vi "Surface Page.vi"() -> ()   [LabVIEW 2020, in "3D Surface.lvclass"]
uses:
  <vilib>/Math Plots/3D Math Plots/3D Surface/3D Surface/3D Surface.lvclass
  <vilib>/Math Plots/3D Math Plots/3D Surface/3D Surface/Typedef/3D Surface Property Array.ctl
  <vilib>/Math Plots/3D Math Plots/3D Surface/3D Surface/Typedef/3D Surface Property.ctl
  <vilib>/Math Plots/3D Math Plots/3D Plot/3D Plot/Typedef/Color Ramp Cluster.ctl
  <vilib>/Math Plots/3D Math Plots/3D Plot/3D Plot/Typedef/Line Type.ctl
  <vilib>/Math Plots/3D Math Plots/3D Plot/3D Plot/Typedef/Dialog State.ctl
  <vilib>/Math Plots/3D Math Plots/3D Plot/3D Plot/Typedef/Temp Scene State.ctl
  <vilib>/Math Plots/3D Math Plots/3D Plot/3D Plot/Typedef/Temp Scene Property Action.ctl
  <vilib>/Math Plots/3D Math Plots/3D Plot/3D Plot/3D Plot.lvclass
panel:
  in  "Draw Normal":bool caption="Draw surface"
  in  "Draw Mesh":bool caption="Draw surface"
  in  "Color Mode":u16(ring) caption="Color mode" items=["Flat Shading", "Interpolated Shading"]
  in  "Antialiasing":bool
  in  "Line Color":u32(colorbox) caption="Line color"
  in  "Line Width":sgl=0.001 caption="Line width" min=0.001 step=1
  in  "Line Style":u16(ring) caption="Line style"
  in  "Draw Surface":bool caption="Draw surface"
  out "Surface Property Out":T1
  in  "Surface Property In":T1
  out "Color Ramp":dbl[][](graph)
  in  "Color Map Style":u16(ring) caption="Color map style" items=["None ", "Shaded", "Color spectrum", "Grey scale", "Custom"]
  in  "YZ Plane Projection":bool caption="YZ plane projection"
  in  "XZ Plane Projection":bool caption="XZ plane projection"
  in  "XY Plane Projection":bool caption="XY plane projection"
  in  "Coordinate System":u16(ring) caption="Coordinate system" items=["Cartesian", "Cylindrical", "Spherical"]
  in  "Plot Opacity":sgl(slide) caption="Plot opacity(%)" min=0 max=100 scale=0.0..100.0
  in  "Plot List":i32(listbox)
  in  "Ramp Edit":bool caption="Ramp edit"
  in  "Move Down":bool
  in  "Move Up":bool
  in  "Delete":bool
  in  "New":bool
  in  "Event Registration":refnum<event-registration>
  # "Surface"
  # "General"
  # "Projection"
  # "Color Ramp"
  # "Surface"
  # "Mesh"
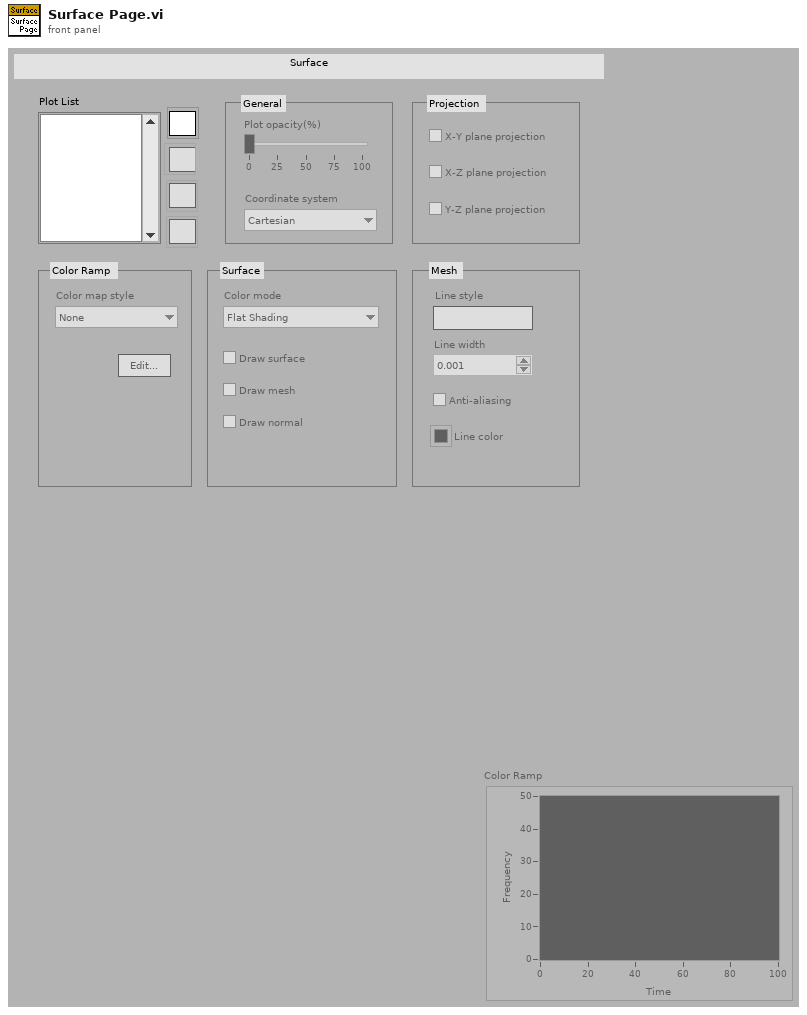
[diagram p1: front panel]
types:
  T1 = typedef "3D Surface.lvclass/3D Surface Property Array.ctl" = T2[]
  T2 = typedef "3D Surface.lvclass/3D Surface Property.ctl" = cluster{"General Property":cluster{"Plot Name":string, "Coordinate System":enum16{"Cartesian", "Cylindrical", "Spherical"}, "Opacity":sgl}, "Projection Property":cluster{"Draw XY":bool, "Draw YZ":bool, "Draw XZ":bool}, "Plot Property":cluster{"Draw Surface":bool, "Draw Mesh":bool, "Draw Normal":bool, "Color Ramp Cluster":T3, "Line Style":T4, "Line Width":sgl, "Line Color":u32, "Antialiasing":bool}, "Surface Property":cluster{"Color Mode":enum16{"Flat Shading", "Interpolated Shading"}}}
  T3 = typedef "3D Plot.lvclass/Color Ramp Cluster.ctl" = cluster{"Color Ramp Style":enum16{"None", "Shaded", "Color spectrum", "Grey scale", "Custom"}, "Color Ramp Array":u32[], "Color Ramp Index":i32[], "Interpolate?":bool, "Logarithm?":bool}
  T4 = typedef "3D Plot.lvclass/Line Type.ctl" = enum16{"None", "Solid", "Dash", "Dot", "Dash Dot"}
  T5 = typedef "3D Plot.lvclass/Dialog State.ctl" = enum16{"Initialize", "Read Porperty", "Write Property", "Idle", "Exit"}
  T6 = typedef "3D Plot.lvclass/Temp Scene State.ctl" = enum16{"Create", "Update Scene", "Get Plot Representation", "Destory"}
  T7 = typedef "3D Plot.lvclass/Temp Scene Property Action.ctl" = enum16{"Graph Property", "Light Property", "Axis Property", "Value Pair Property", "Format Property", "Cursor Property", "Plot Specific Property"}
  T8 = typedef "3D Plot.lvclass/Multiplot Representation.ctl" = cluster{"Plot Represention Array":T9[], "Max Range":T10}
  T9 = typedef "3D Plot.lvclass/Plot Representation.ctl" = cluster{"Plot ID":i32, "Plot Range":T10, "Mesh Data":T11, "Dimension":cluster{"X Dimension":i32, "Y Dimension":i32}, "Ramp Range":T10}
  T10 = typedef "3D Plot.lvclass/Range Clusters.ctl" = cluster{"X Range":cluster{"Max X":sgl, "Min X":sgl}, "Y Range":cluster{"Max Y":sgl, "Min Y":sgl}, "Z Range":cluster{"Max Z":sgl, "Min Z":sgl}}
  T11 = typedef "3D Plot.lvclass/Mesh Data.ctl" = cluster{"Index Array":u32[], "Vertex Array":cluster{"X":sgl, "Y":sgl, "Z":sgl}[], "Normal Array":cluster{"X":sgl, "Y":sgl, "Z":sgl}[], "Color Index Array":i32[]}
  T12 = enum16{"None", "Shaded", "Color spectrum", "Grey scale", "Custom"}
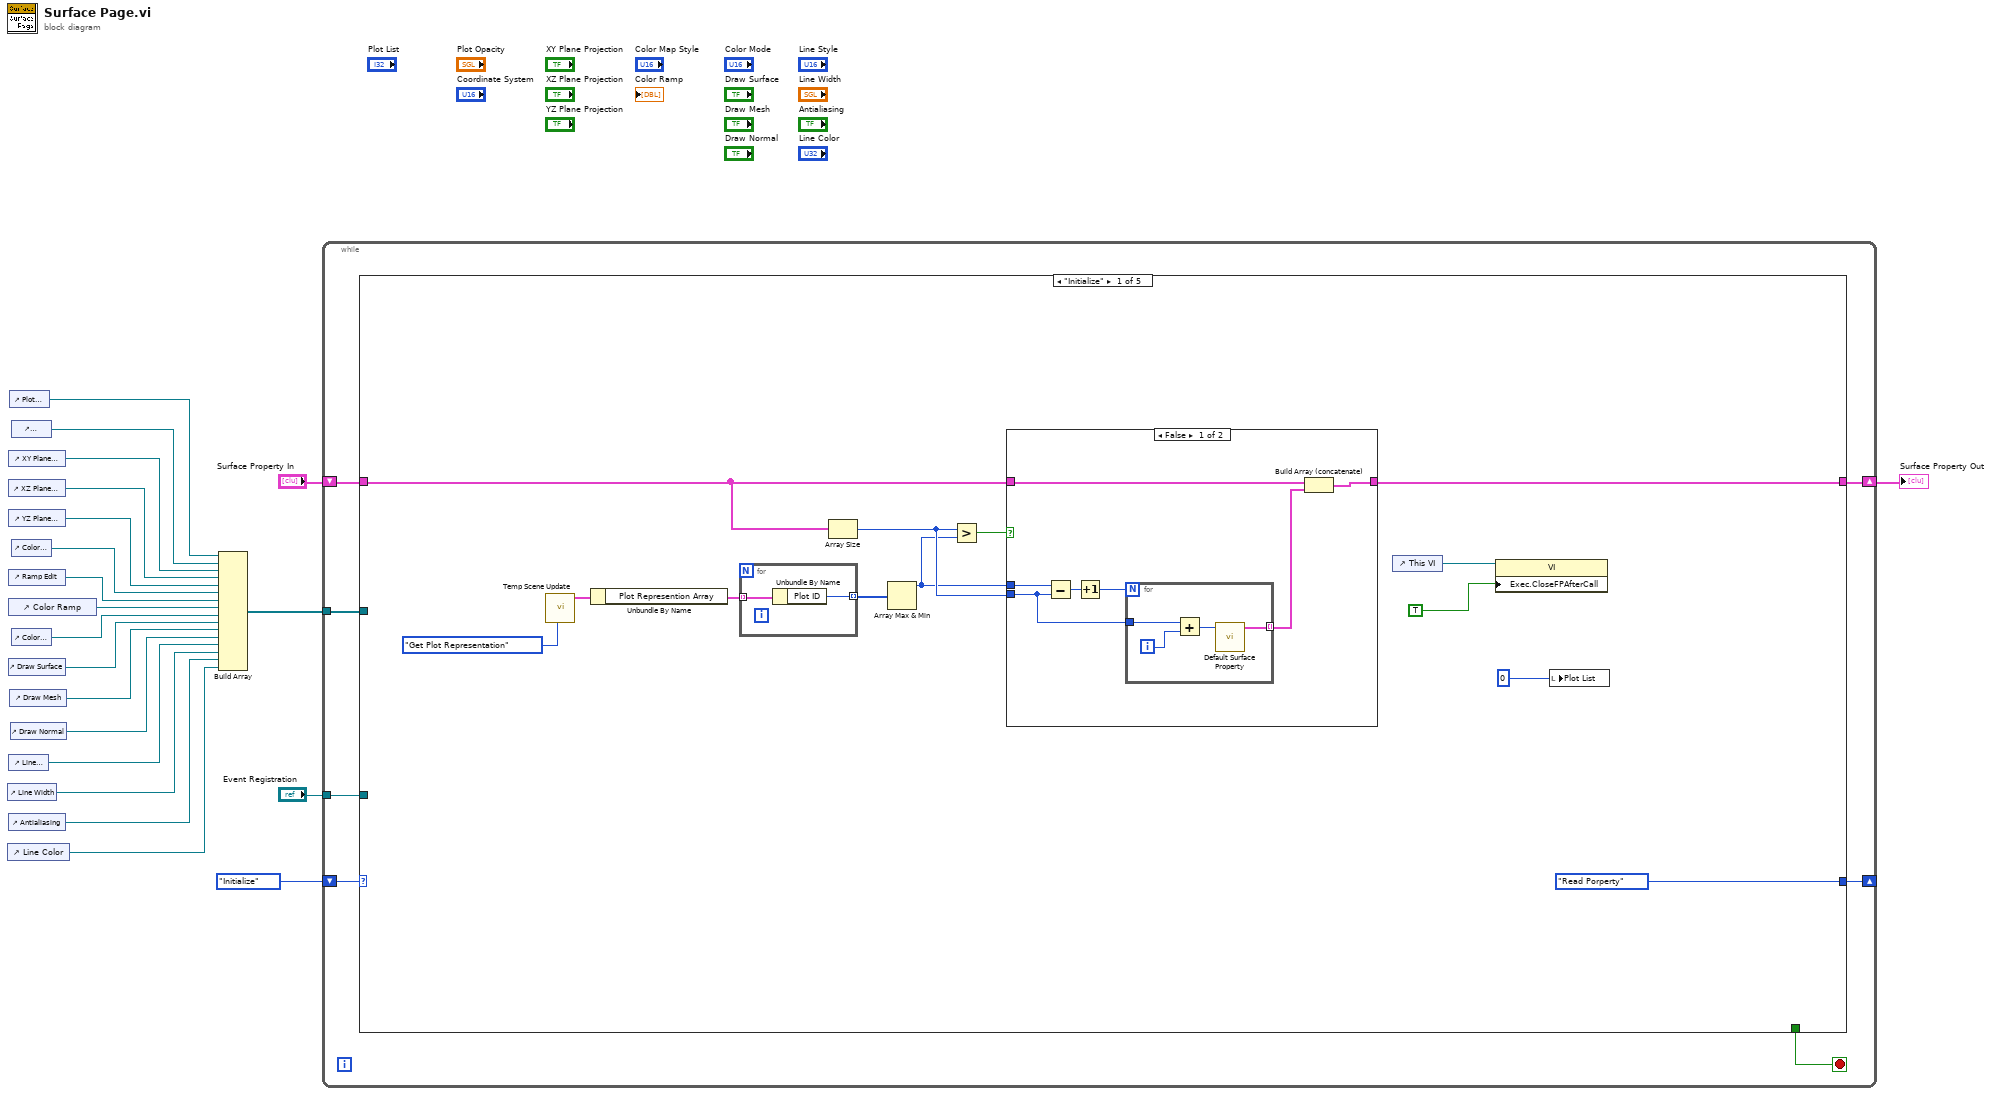
[diagram p0: block diagram]
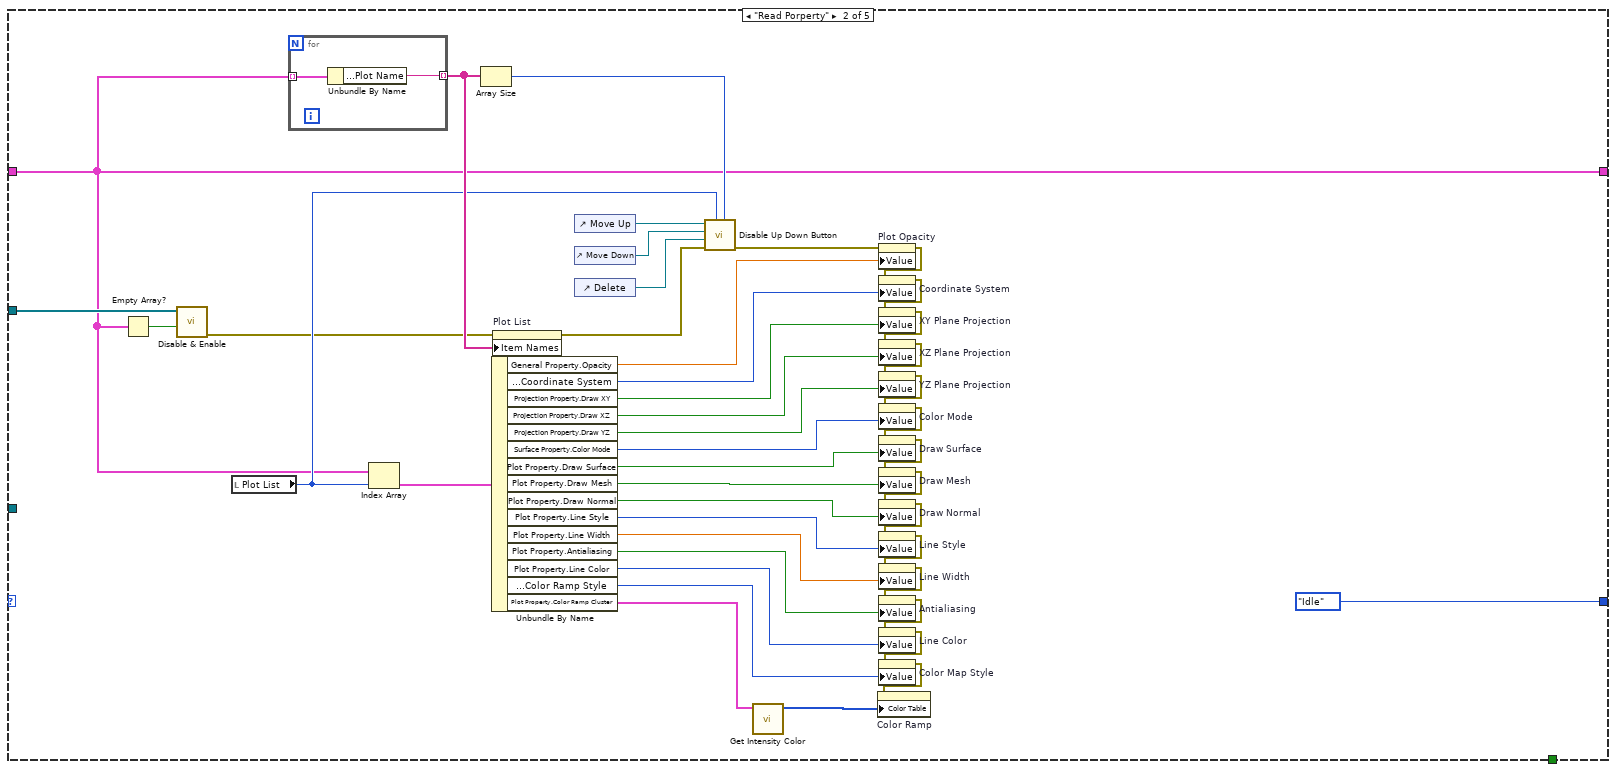
[diagram p3: hidden frame]
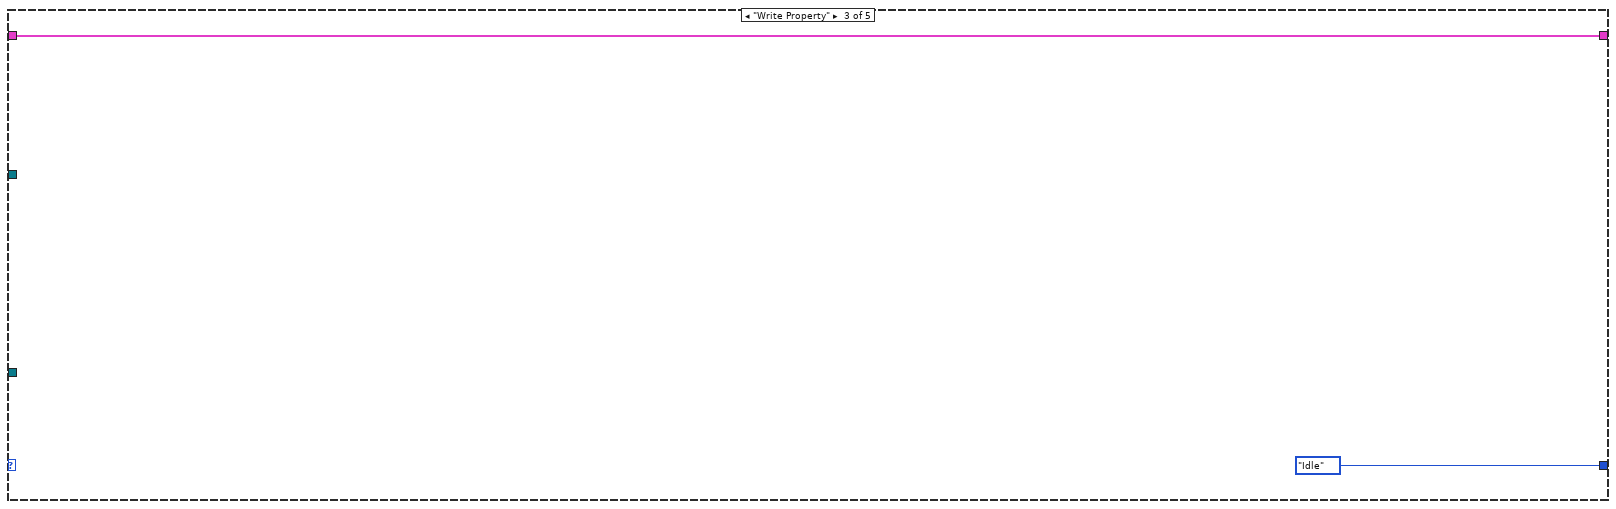
[diagram p4: hidden frame]
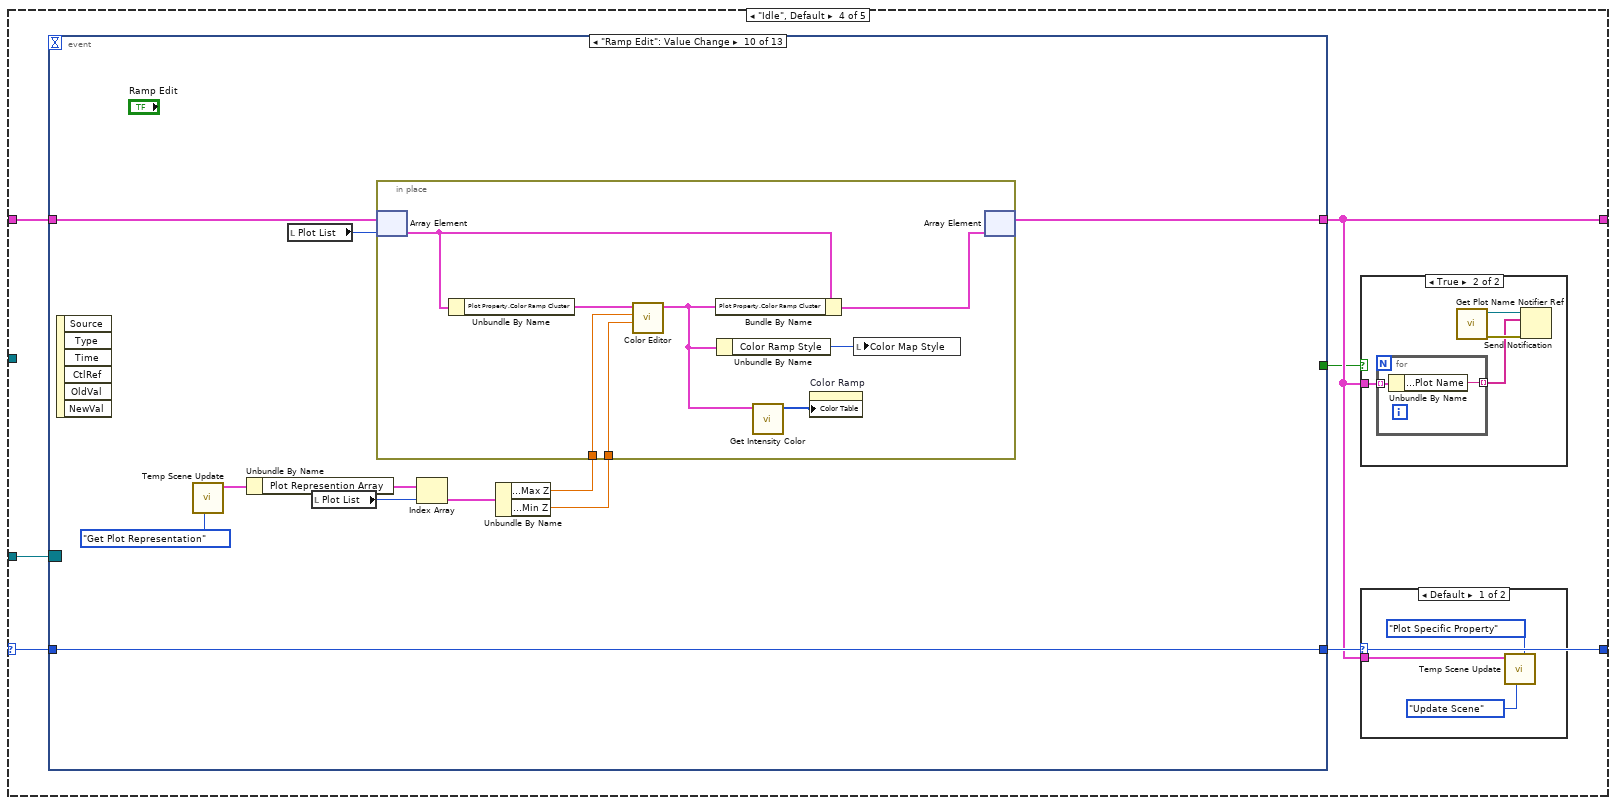
[diagram p5: hidden frame]
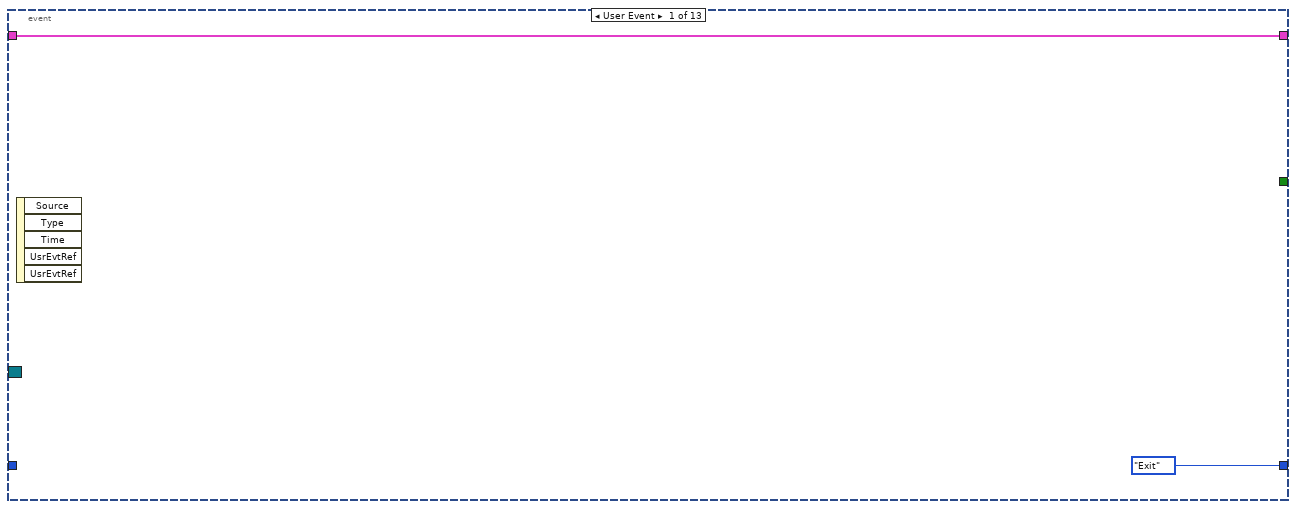
[diagram p8: hidden frame]
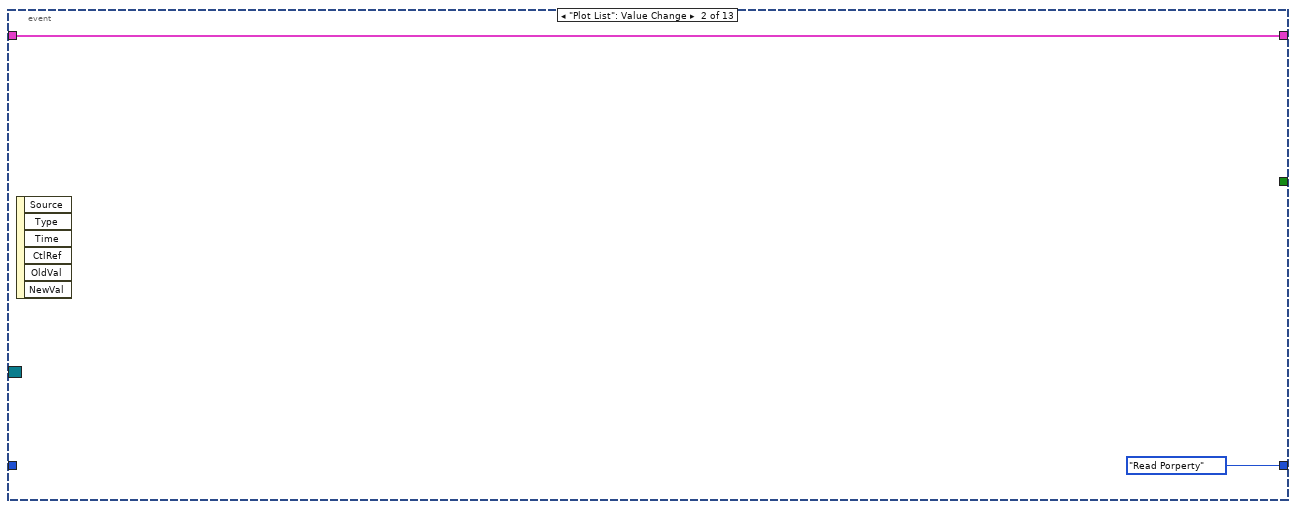
[diagram p9: hidden frame]
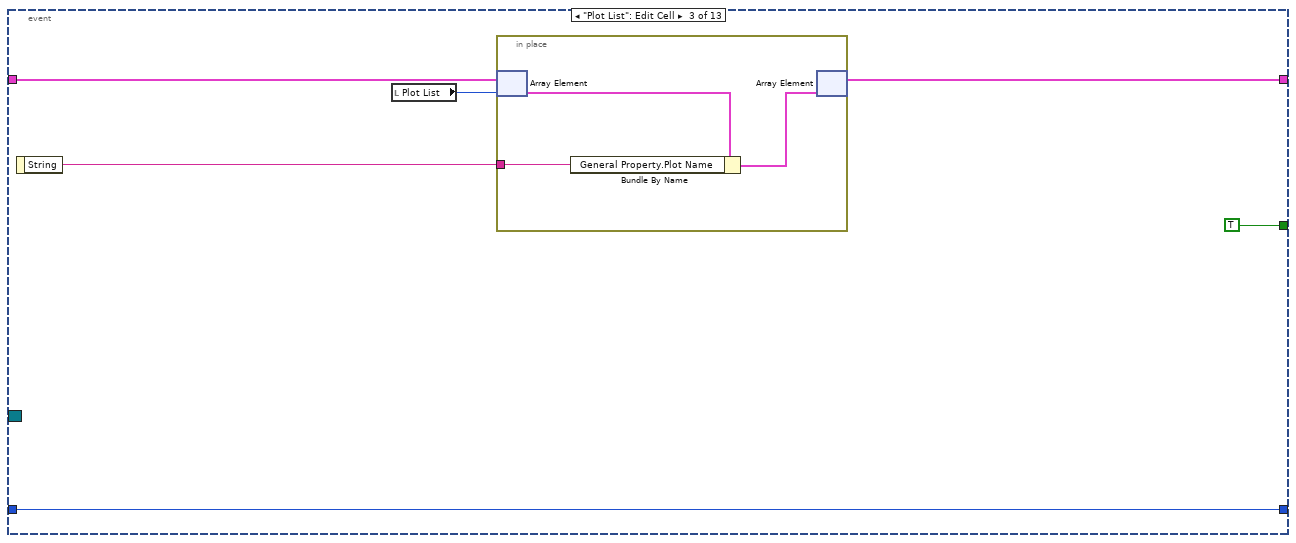
[diagram p10: hidden frame]
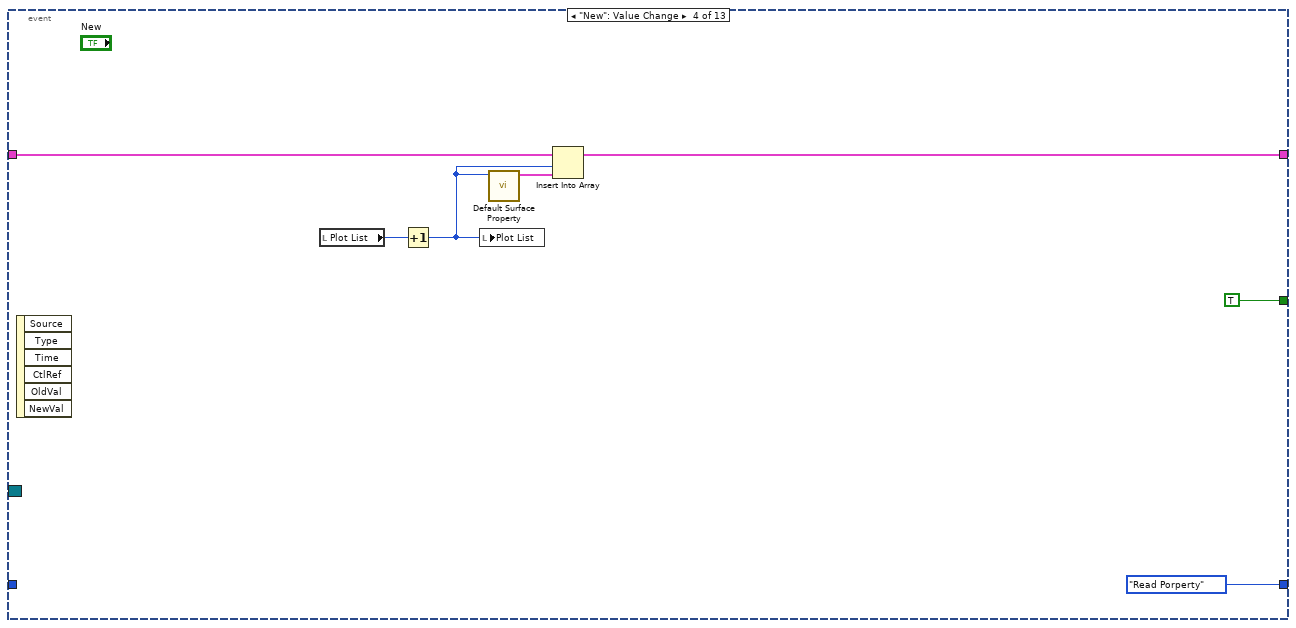
[diagram p11: hidden frame]
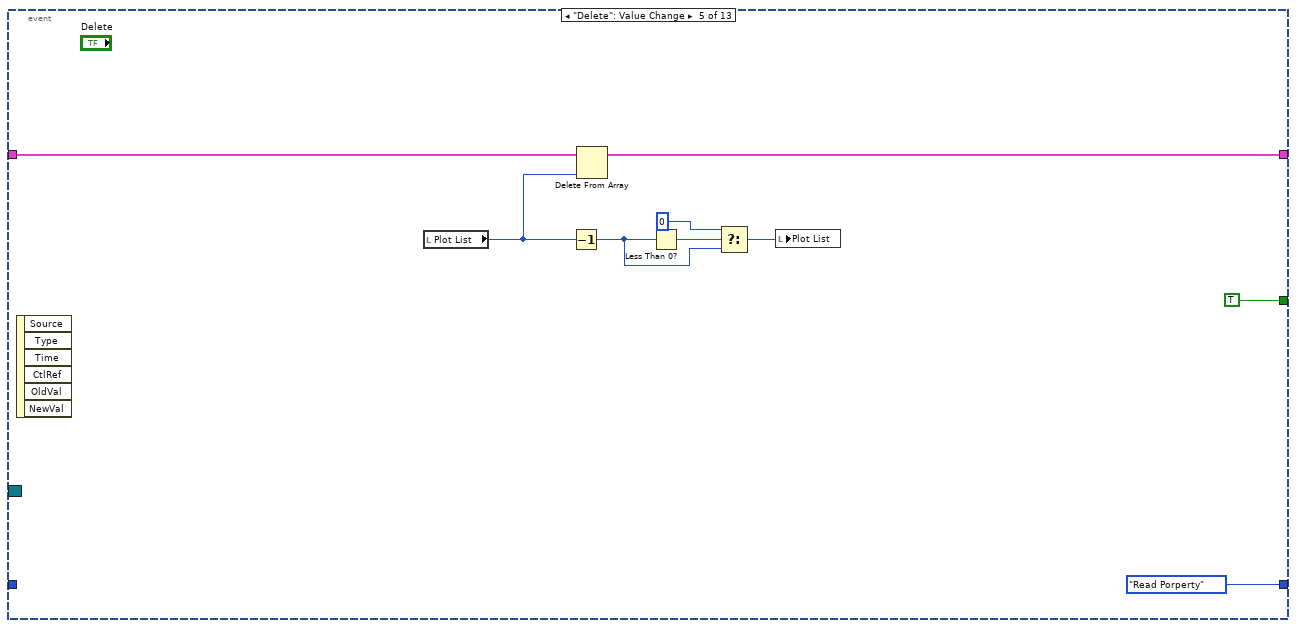
[diagram p12: hidden frame]
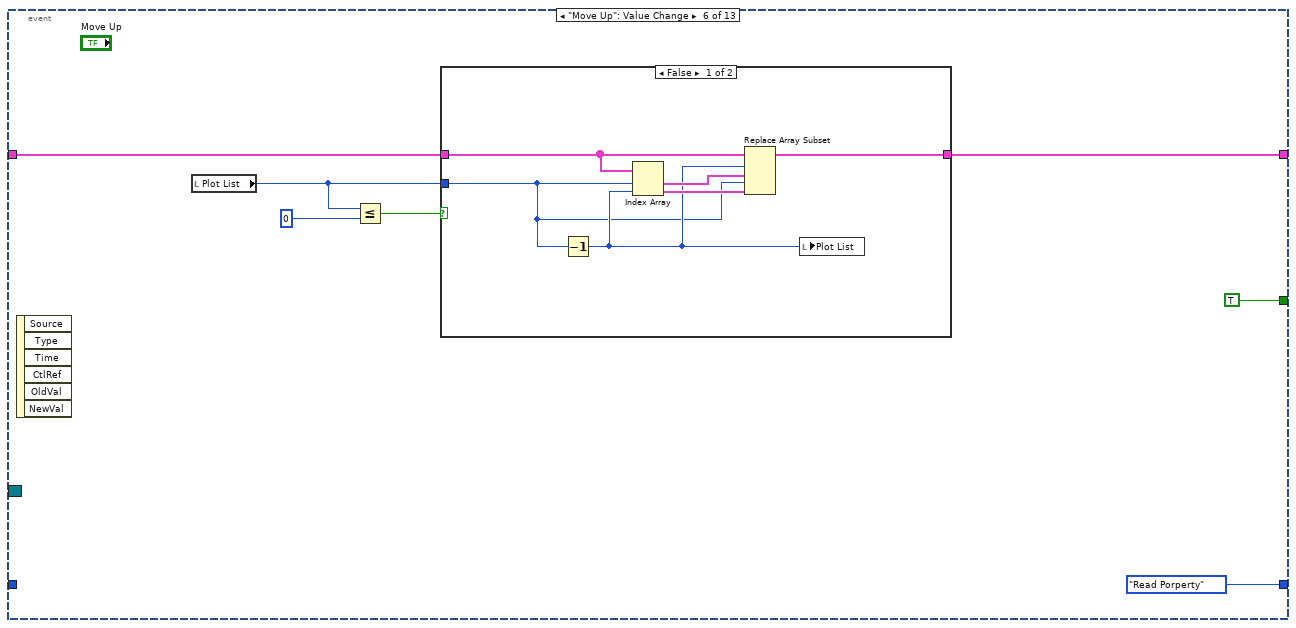
[diagram p13: hidden frame]
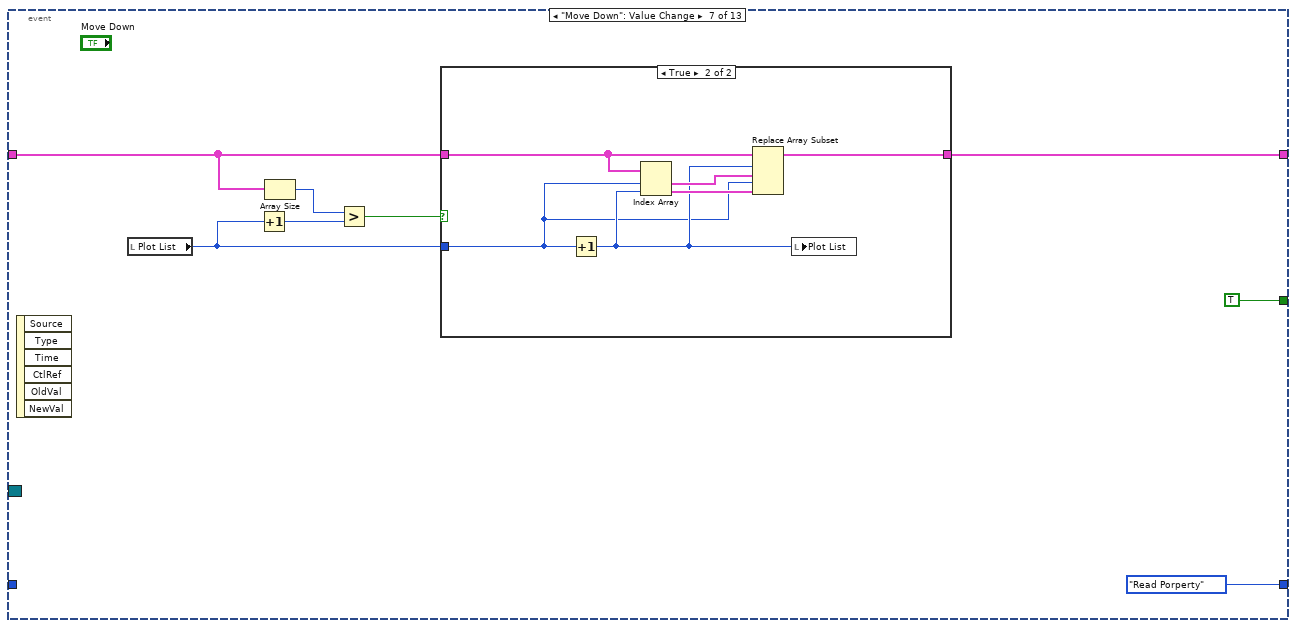
[diagram p15: hidden frame]
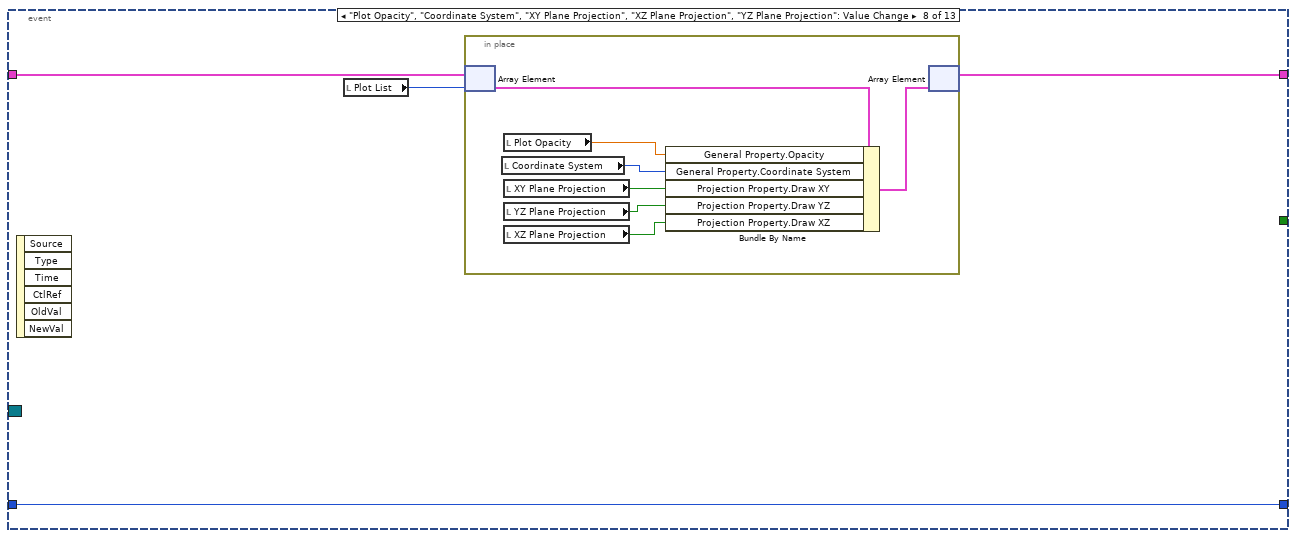
[diagram p17: hidden frame]
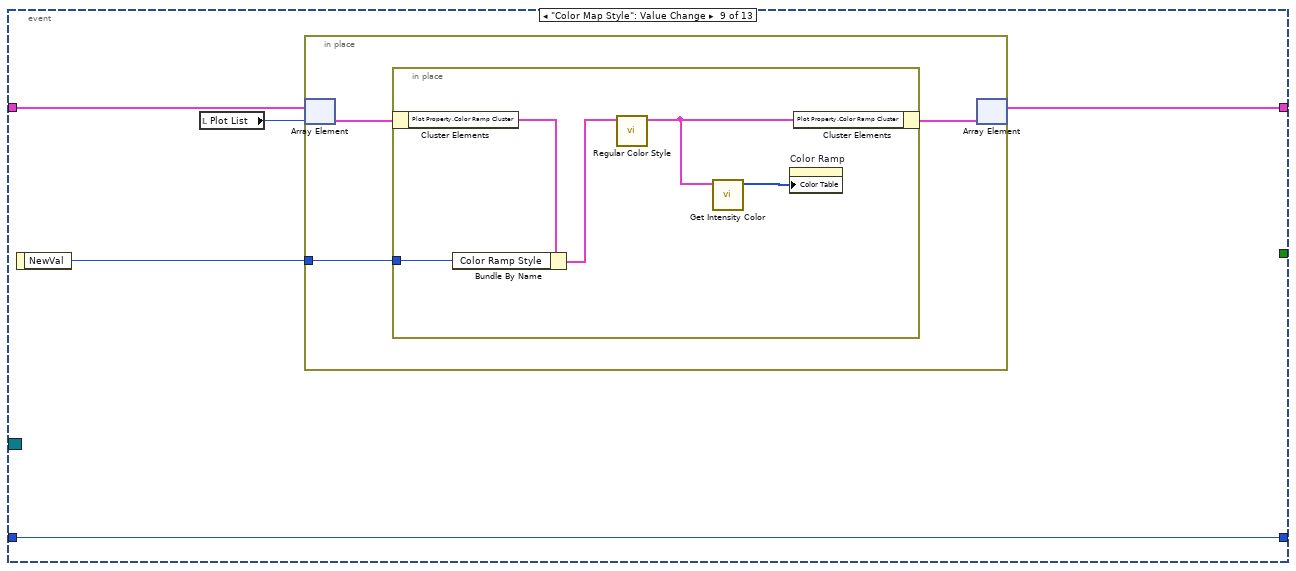
[diagram p18: hidden frame]
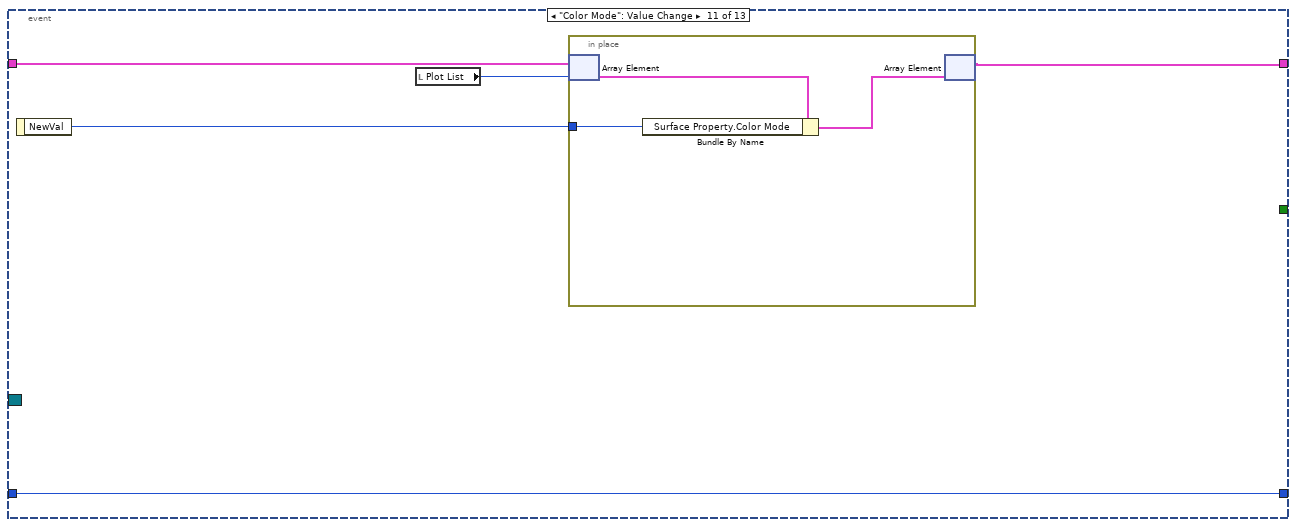
[diagram p19: hidden frame]
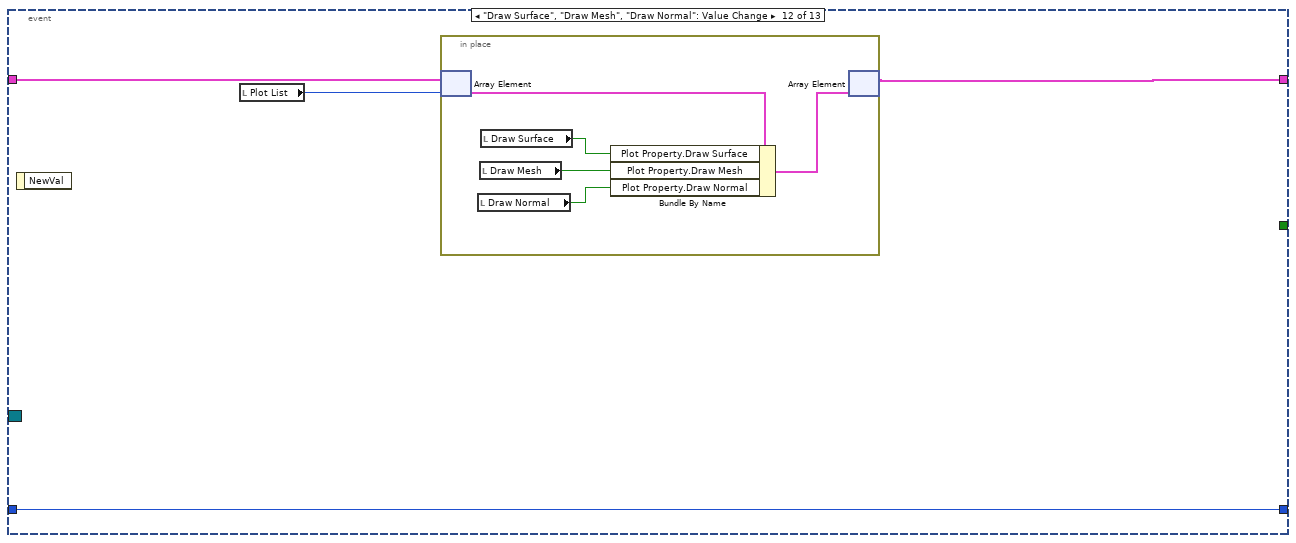
[diagram p20: hidden frame]
diagram:
  n1 = control-ref of="Line Width"() -> (w6:refnum<vi>)
  n2 = control-ref of="Line Color"() -> (w4:refnum<vi>)
  n3 = control-ref of="XY Plane Projection"() -> (w15:refnum<vi>)
  n4 = control-ref of="XZ Plane Projection"() -> (w14:refnum<vi>)
  n5 = control-ref of="YZ Plane Projection"() -> (w13:refnum<vi>)
  n6 = control-ref of="Ramp Edit"() -> (w11:refnum<vi>)
  n7 = control-ref of="Color Ramp"() -> (w10:refnum<vi>)
  n8 = control-ref of="Draw Surface"() -> (w8:refnum<vi>)
  n9 = control-ref of="Line Style"() -> (w7:refnum<vi>)
  n10 = control-ref of="Antialiasing"() -> (w5:refnum<vi>)
  n11 = control-ref of="Plot Opacity"() -> (w17:refnum<vi>)
  n12 = control-ref of="Draw Mesh"() -> (w1:refnum<vi>)
  n13 = control-ref of="Draw Normal"() -> (w2:refnum<vi>)
  n14 = control-ref of="Coordinate System"() -> (w16:refnum<vi>)
  n15 = control-ref of="Color Map Style"() -> (w12:refnum<vi>)
  n16 = control-ref of="Color Mode"() -> (w9:refnum<vi>)
  n17 = Build Array(w17, w16, w15, w14, w13, w12, w11, w10, w9, w8, w1, w2, w7, w6, w5, w4) -> (w3:refnum<vi>[])
  n18 = while {
    shift-right: [w27] -> w18
    shift-left: "Surface Property In" -> [w28]
    shift-right: [w23] -> _
    shift-left: Dialog_State."Initialize" -> [w26]
    tunnel: "Event Registration" -> [w24]
    tunnel: w3 -> [w22]
    stop <- w25 stop-if-true
    n19 = case shown="\"Initialize\"" w26 {
      selector: w26 -> [_ _ _ w107 _]
      tunnel: w28 -> [w33 w88 w102 w109 w247]
      tunnel: [w34 w88 w102 w105 w247] -> w27
      tunnel: [Dialog_State."Read Porperty" Dialog_State."Idle" Dialog_State."Idle" w106 Dialog_State."Exit"] -> w23
      tunnel: [_ _ _ _ TRUE] -> w25
      tunnel: w24 -> [_ _ _ w108 _]
      tunnel: w22 -> [_ w89 _ _ _]
      frame "Initialize" {
        n20 = call <vilib>:"Temp Scene Update.vi"("State"=Temp_Scene_State."Get Plot Representation") -> ("Multiplot Representation"=w36:T8)  [unwired: 5 in, 5 out]
        n21 = Unbundle By Name(w36) -> ("Plot Represention Array"=w29:T9[])
        n22 = for {
          tunnel: w29 -> [w55] mode=indexing
          tunnel: [w54] -> w35 mode=indexing
          n23 = Unbundle By Name(w55) -> ("Plot ID"=w54:i32)
        }
        n24 = Array Size(array=w33) -> (size(s)=w31:i32)
        n25 = Array Max & Min(array=w35) -> (max value=w30:i32)  [unwired: 3 out]
        n26 = Greater?(x=w31, y=w30) -> (0:w32:bool)
        n27 = case shown="False" w32 {
          tunnel: [w46 w53] -> w34
          tunnel: w33 -> [w48 w53]
          tunnel: w31 -> [w42 _]
          tunnel: w30 -> [w43 _]
          frame False {
            n28 = Subtract(x=w43, y=w42) -> (x-y=w45:i32)
            n29 = Increment(x=w45) -> (x+1=w44:i32)
            n30 = for {
              N: w44 -> [_]
              tunnel: w42 -> [w50]
              tunnel: [w49] -> w47 mode=indexing
              i -> [w51]
              n31 = Add(x=w50, y=w51) -> (x+y=w52:i32)
              n32 = call <vilib>:"Default Surface Property.vi"("Plot ID"=w52) -> ("Default Property"=w49:T2)  [unwired: 10 out]
            }
            n33 = Build Array (concatenate)(w48, w47) -> (w46:T1)
          }
          frame True {
          }
        }
        n34 = control-ref of="This VI"() -> (w40:refnum<vi>)
        n35 = property class="VI"(reference=w40, "Exec.CloseFPAfterCall"=TRUE ("Execution:Close After Call")) -> ()  [unwired: 1 in, 2 out]
        n36 = local write "Plot List"(0 ("Plot List")) -> ()
      }
      frame "Read Porperty" {
        n37 = Empty Array?(array=w88) -> (empty?=w87:bool)
        n38 = call <vilib>:"Disable & Enable.vi"("Disabled?"=w87, "Control Ref Array"=w89) -> ("error out"=w86:errorcluster)  [unwired: 1 in, 8 out]
        n39 = local read "Plot List"() -> (w93:i32)
        n40 = for {
          tunnel: w88 -> [w101] mode=indexing
          tunnel: [w100] -> w95 mode=indexing
          n41 = Unbundle By Name(w101) -> ("General Property.Plot Name"=w100:string)
        }
        n42 = Index Array(array=w88, index=w93) -> (element=w98:T2)
        n43 = Array Size(array=w95) -> (size(s)=w96:i32)
        n44 = Unbundle By Name(w98) -> ("General Property.Opacity"=w85:sgl, "General Property.Coordinate System"=w84:enum16{"Cartesian", "Cylindrical", "Spherical"}, "Projection Property.Draw XY"=w83:bool, "Projection Property.Draw XZ"=w82:bool, "Projection Property.Draw YZ"=w81:bool, "Surface Property.Color Mode"=w80:enum16{"Flat Shading", "Interpolated Shading"}, "Plot Property.Draw Surface"=w79:bool, "Plot Property.Draw Mesh"=w78:bool, "Plot Property.Draw Normal"=w77:bool, "Plot Property.Line Style"=w76:T4, "Plot Property.Line Width"=w75:sgl, "Plot Property.Antialiasing"=w74:bool, "Plot Property.Line Color"=w73:u32, "Plot Property.Color Ramp Cluster.Color Ramp Style"=w72:T12, "Plot Property.Color Ramp Cluster"=w56:T3)
        n45 = property on="Plot List" class="LstBox (strict)"(error in=w86, "Item Names"=w95) -> (error out=w94:errorcluster)  [unwired: 1 in, 1 out]
        n46 = control-ref of="Move Up"() -> (w90:refnum<vi>)
        n47 = control-ref of="Move Down"() -> (w91:refnum<vi>)
        n48 = control-ref of="Delete"() -> (w92:refnum<vi>)
        n49 = call <vilib>:"Disable Up Down Button.vi"("Length"=w96, "Index"=w93, "error in (no error)"=w94, "Delete Ref"=w92, "Move Down Ref"=w91, "Move Up Ref"=w90) -> ("error out"=w71:errorcluster)  [unwired: 5 out]
        n50 = call <vilib>:"Get Intensity Color.vi"("Color Ramp Cluster"=w56) -> ("Intensity Color"=w97:u32[])  [unwired: 4 in, 6 out]
        n51 = property on="Plot Opacity" class="Slide (strict)"(error in=w71, "Value"=w85) -> (error out=w70:errorcluster)  [unwired: 1 in, 1 out]
        n52 = property on="Coordinate System" class="Ring (strict)"(error in=w70, "Value"=w84) -> (error out=w69:errorcluster)  [unwired: 1 in, 1 out]
        n53 = property on="XY Plane Projection" class="Bool (strict)"(error in=w69, "Value"=w83) -> (error out=w68:errorcluster)  [unwired: 1 in, 1 out]
        n54 = property on="XZ Plane Projection" class="Bool (strict)"(error in=w68, "Value"=w82) -> (error out=w67:errorcluster)  [unwired: 1 in, 1 out]
        n55 = property on="YZ Plane Projection" class="Bool (strict)"(error in=w67, "Value"=w81) -> (error out=w66:errorcluster)  [unwired: 1 in, 1 out]
        n56 = property on="Color Mode" class="Ring (strict)"(error in=w66, "Value"=w80) -> (error out=w65:errorcluster)  [unwired: 1 in, 1 out]
        n57 = property on="Draw Surface" class="Bool (strict)"(error in=w65, "Value"=w79) -> (error out=w64:errorcluster)  [unwired: 1 in, 1 out]
        n58 = property on="Draw Mesh" class="Bool (strict)"(error in=w64, "Value"=w78) -> (error out=w63:errorcluster)  [unwired: 1 in, 1 out]
        n59 = property on="Draw Normal" class="Bool (strict)"(error in=w63, "Value"=w77) -> (error out=w62:errorcluster)  [unwired: 1 in, 1 out]
        n60 = property on="Line Style" class="Ring (strict)"(error in=w62, "Value"=w76) -> (error out=w61:errorcluster)  [unwired: 1 in, 1 out]
        n61 = property on="Line Width" class="DigNum (strict)"(error in=w61, "Value"=w75) -> (error out=w60:errorcluster)  [unwired: 1 in, 1 out]
        n62 = property on="Antialiasing" class="Bool (strict)"(error in=w60, "Value"=w74) -> (error out=w59:errorcluster)  [unwired: 1 in, 1 out]
        n63 = property on="Line Color" class="ColBox"(error in=w59, "Value"=w73) -> (error out=w58:errorcluster)  [unwired: 1 in, 1 out]
        n64 = property on="Color Map Style" class="Ring (strict)"(error in=w58, "Value"=w72) -> (error out=w57:errorcluster)  [unwired: 1 in, 1 out]
        n65 = property on="Color Ramp" class="IntGraph (strict)"(error in=w57, "Color Table"=w97) -> ()  [unwired: 1 in, 2 out]
      }
      frame "Write Property" {
      }
      frame "Idle", Default {
        n66 = event shown="[9] \"Ramp Edit\": Value Change" {
          selector: w108 -> [_ _ _ _ _ _ _ _ _ _ _ _ _]
          dyn-events: _ -> [_ _ _ _ _ _ _ _ _ _ _ _ _]
          timeout: _ -> [_ _ _ _ _ _ _ _ _ _ _ _ _]
          tunnel: w109 -> [w120 w122 w126 w136 w145 w154 w165 w178 w189 w209 w222 w229 w238]
          tunnel: [w120 w122 w125 w135 w146 w153 w169 w177 w188 w208 w221 w228 w237] -> w105
          tunnel: [Dialog_State."Exit" Dialog_State."Read Porperty" w124 Dialog_State."Read Porperty" Dialog_State."Read Porperty" Dialog_State."Read Porperty" Dialog_State."Read Porperty" w180 w192 w211 w224 w230 w239] -> w106
          tunnel: w107 -> [_ _ w124 _ _ _ _ w180 w192 w211 w224 w230 w239]
          tunnel: [_ _ TRUE TRUE TRUE TRUE TRUE _ _ _ _ _ _] -> w104
          event User Event {
            n67 = event-data() -> ()  [unwired: 6 out]
          }
          event "Plot List": Value Change {
            n68 = event-data() -> ()  [unwired: 7 out]
          }
          event "Plot List": Edit Cell {
            n69 = event-data() -> ("String"=w127:string)  [unwired: 1 out]
            n70 = local read "Plot List"() -> (w128:i32)
            n71 = in-place {
              in-place-border: w127 -> [w129]
              n72 = in-place-array #1(w126, w128) -> (w131:T2)
              n73 = Bundle By Name(cluster=w131, "General Property.Plot Name"=w129) -> (w130:T2)
              n74 = in-place-array #1(w130) -> (w125:T1)  [unwired: 1 out]
            }
          }
          event "New": Value Change {
            n75 = event-data() -> ()  [unwired: 7 out]
            n76 = local read "Plot List"() -> (w137:i32)
            n77 = Increment(x=w137) -> (x+1=w132:i32)
            n78 = local write "Plot List"(w132) -> ()
            n79 = call <vilib>:"Default Surface Property.vi"("Plot ID"=w132) -> ("Default Property"=w133:T2)  [unwired: 10 out]
            n80 = Insert Into Array(array=w136, index=w132, new element=w133) -> (w135:T1)
          }
          event "Delete": Value Change {
            n81 = event-data() -> ()  [unwired: 7 out]
            n82 = local read "Plot List"() -> (w141:i32)
            n83 = Decrement(x=w141) -> (x-1=w142:i32)
            n84 = Delete From Array(array=w145, index=w141) -> (array with subset deleted=w146:T1)  [unwired: 1 in, 1 out]
            n85 = Less Than 0?(x=w142) -> (x < 0?=w144:bool)
            n86 = Select(t=0, s=w144, f=w142) -> (s? t:f=w140:i32)
            n87 = local write "Plot List"(w140) -> ()
          }
          event "Move Up": Value Change {
            n88 = event-data() -> ()  [unwired: 7 out]
            n89 = local read "Plot List"() -> (w149:i32)
            n90 = Less Or Equal?(x=w149, y=0) -> (x <= y?=w150:bool)
            n91 = case shown="False" w150 {
              tunnel: w154 -> [w158 w161]
              tunnel: [w157 w161] -> w153
              tunnel: w149 -> [w155 _]
              frame False {
                n92 = Decrement(x=w155) -> (x-1=w156:i32)
                n93 = Index Array(array=w158, index #1=w155, index #2=w156) -> (element #1=w160:T2, element #2=w159:T2)
                n94 = Replace Array Subset(array=w158, new element #1=w160, index #1=w156, new element #2=w159, index #2=w155) -> (w157:T1)
                n95 = local write "Plot List"(w156) -> ()
              }
              frame True {
                # "List value is less or equal to 0.\nThe active item is in the top of the list."
              }
            }
          }
          event "Move Down": Value Change {
            n96 = event-data() -> ()  [unwired: 7 out]
            n97 = local read "Plot List"() -> (w163:i32)
            n98 = Increment(x=w163) -> (x+1=w166:i32)
            n99 = Array Size(array=w165) -> (size(s)=w167:i32)
            n100 = Greater?(x=w167, y=w166) -> (0:w164:bool)
            n101 = case shown="True" w164 {
              tunnel: w165 -> [w170 w173]
              tunnel: [w170 w172] -> w169
              tunnel: w163 -> [_ w171]
              frame False {
                # "List value +1 is not less array length.\nThe active item is in the buttom of the list."
              }
              frame True {
                n102 = Increment(x=w171) -> (x+1=w174:i32)
                n103 = Index Array(array=w173, index #1=w171, index #2=w174) -> (element #1=w176:T2, element #2=w175:T2)
                n104 = Replace Array Subset(array=w173, new element #1=w176, index #1=w174, new element #2=w175, index #2=w171) -> (w172:T1)
                n105 = local write "Plot List"(w174) -> ()
              }
            }
          }
          event "Plot Opacity", "Coordinate System", "XY Plane Projection", "XZ Plane Projection", "YZ Plane Projection": Value Change {
            n106 = event-data() -> ()  [unwired: 7 out]
            n107 = local read "Plot List"() -> (w179:i32)
            n108 = in-place {
              n109 = in-place-array #2(w178, w179) -> (w183:T2)
              n110 = local read "Coordinate System"() -> (w181:u16)
              n111 = local read "Plot Opacity"() -> (w187:sgl)
              n112 = local read "XY Plane Projection"() -> (w186:bool)
              n113 = local read "YZ Plane Projection"() -> (w184:bool)
              n114 = local read "XZ Plane Projection"() -> (w185:bool)
              n115 = Bundle By Name(cluster=w183, "General Property.Opacity"=w187, "General Property.Coordinate System"=w181, "Projection Property.Draw XY"=w186, "Projection Property.Draw YZ"=w184, "Projection Property.Draw XZ"=w185) -> (w182:T2)
              n116 = in-place-array #2(w182) -> (w177:T1)  [unwired: 1 out]
            }
          }
          event "Color Map Style": Value Change {
            n117 = event-data() -> ("NewVal"=w190:u16)  [unwired: 1 out]
            n118 = local read "Plot List"() -> (w191:i32)
            n119 = in-place {
              in-place-border: w190 -> [w194]
              n120 = in-place-array #3(w189, w191) -> (w195:T2)
              n121 = in-place {
                in-place-border: w194 -> [w199]
                n122 = in-place-cluster #4(w195) -> ("Plot Property.Color Ramp Cluster"=w200:T3)
                n123 = Bundle By Name(cluster=w200, "Color Ramp Style"=w199) -> (w198:T3)
                n124 = call <vilib>:"Regular Color Style.vi"("Color Ramp Cluster in"=w198) -> ("Color Ramp Cluster out"=w196:T3)  [unwired: 10 in]
                n125 = call <vilib>:"Get Intensity Color.vi"("Color Ramp Cluster"=w196) -> ("Intensity Color"=w197:u32[])  [unwired: 4 in, 6 out]
                n126 = property on="Color Ramp" class="IntGraph (strict)"("Color Table"=w197) -> ()  [unwired: 2 in, 2 out]
                n127 = in-place-cluster #4("Plot Property.Color Ramp Cluster"=w196) -> (w193:T2)
              }
              n128 = in-place-array #3(w193) -> (w188:T1)  [unwired: 1 out]
            }
          }
          event "Ramp Edit": Value Change {
            n129 = event-data() -> ()  [unwired: 7 out]
            n130 = call <vilib>:"Temp Scene Update.vi"("State"=Temp_Scene_State."Get Plot Representation") -> ("Multiplot Representation"=w204:T8)  [unwired: 5 in, 5 out]
            n131 = Unbundle By Name(w204) -> ("Plot Represention Array"=w201:T9[])
            n132 = local read "Plot List"() -> (w210:i32)
            n133 = local read "Plot List"() -> (w207:i32)
            n134 = Index Array(array=w201, index=w207) -> (element=w206:T9)
            n135 = Unbundle By Name(w206) -> ("Plot Range.Z Range.Max Z"=w203:sgl, "Plot Range.Z Range.Min Z"=w202:sgl)
            n136 = in-place {
              in-place-border: w203 -> [w215]
              in-place-border: w202 -> [w214]
              n137 = in-place-array #5(w209, w210) -> (w218:T2)
              n138 = Unbundle By Name(w218) -> ("Plot Property.Color Ramp Cluster"=w216:T3)
              n139 = call <vilib>:"Color Editor.vi"("Min"=w214, "Max"=w215, "Color Ramp Cluster in"=w216) -> ("Color Ramp Cluster out"=w213:T3)  [unwired: 3 in, 5 out]
              n140 = Bundle By Name(cluster=w218, "Plot Property.Color Ramp Cluster"=w213) -> (w219:T2)
              n141 = Unbundle By Name(w213) -> ("Color Ramp Style"=w212:T12)
              n142 = call <vilib>:"Get Intensity Color.vi"("Color Ramp Cluster"=w213) -> ("Intensity Color"=w217:u32[])  [unwired: 4 in, 6 out]
              n143 = property on="Color Ramp" class="IntGraph (strict)"("Color Table"=w217) -> ()  [unwired: 2 in, 2 out]
              n144 = local write "Color Map Style"(w212) -> ()
              n145 = in-place-array #5(w219) -> (w208:T1)  [unwired: 1 out]
            }
          }
          event "Color Mode": Value Change {
            n146 = event-data() -> ("NewVal"=w220:u16)  [unwired: 1 out]
            n147 = local read "Plot List"() -> (w223:i32)
            n148 = in-place {
              in-place-border: w220 -> [w225]
              n149 = in-place-array #6(w222, w223) -> (w227:T2)
              n150 = Bundle By Name(cluster=w227, "Surface Property.Color Mode"=w225) -> (w226:T2)
              n151 = in-place-array #6(w226) -> (w221:T1)  [unwired: 1 out]
            }
          }
          event "Draw Surface", "Draw Mesh", "Draw Normal": Value Change {
            n152 = event-data() -> ()  [unwired: 2 out]
            n153 = local read "Plot List"() -> (w231:i32)
            n154 = in-place {
              n155 = in-place-array #7(w229, w231) -> (w236:T2)
              n156 = local read "Draw Normal"() -> (w232:bool)
              n157 = local read "Draw Mesh"() -> (w233:bool)
              n158 = local read "Draw Surface"() -> (w234:bool)
              n159 = Bundle By Name(cluster=w236, "Plot Property.Draw Surface"=w234, "Plot Property.Draw Mesh"=w233, "Plot Property.Draw Normal"=w232) -> (w235:T2)
              n160 = in-place-array #7(w235) -> (w228:T1)  [unwired: 1 out]
            }
          }
          event "Line Style", "Line Width", "Antialiasing", "Line Color": Value Change {
            n161 = event-data() -> ()  [unwired: 2 out]
            n162 = local read "Plot List"() -> (w240:i32)
            n163 = in-place {
              n164 = in-place-array #8(w238, w240) -> (w246:T2)
              n165 = local read "Antialiasing"() -> (w243:bool)
              n166 = local read "Line Color"() -> (w244:u32)
              n167 = local read "Line Width"() -> (w242:sgl)
              n168 = local read "Line Style"() -> (w241:u16)
              n169 = Bundle By Name(cluster=w246, "Plot Property.Line Style"=w241, "Plot Property.Line Width"=w242, "Plot Property.Antialiasing"=w243, "Plot Property.Line Color"=w244) -> (w245:T2)
              n170 = in-place-array #8(w245) -> (w237:T1)  [unwired: 1 out]
            }
          }
        }
        n171 = case shown="True" w104 {
          tunnel: w105 -> [_ w110]
          frame False {
          }
          frame True {
            n172 = for {
              tunnel: w110 -> [w115] mode=indexing
              tunnel: [w114] -> w111 mode=indexing
              n173 = Unbundle By Name(w115) -> ("General Property.Plot Name"=w114:string)
            }
            n174 = call <vilib>:"Get Plot Name Notifier Ref.vi"() -> ("error out"=w113:errorcluster, "Plot Names Notifier Ref"=w112:refnum<notifier>)  [unwired: 1 in, 9 out]
            n175 = Send Notification(notification=w111, notifier=w112, error in (no error)=w113) -> ()  [unwired: 2 out]
          }
        }
        n176 = case shown="Default" w106 {
          tunnel: w105 -> [w118 _]
          frame Default {
            n177 = call <vilib>:"Temp Scene Update.vi"("Property Name"=Temp_Scene_Property_Action."Plot Specific Property", "State"=Temp_Scene_State."Update Scene", "Property In"=w118) -> ()  [unwired: 3 in, 6 out]
          }
          frame "Exit" {
          }
        }
      }
      frame "Exit" {
      }
    }
  }
  "Surface Property Out" <- w18
